vi "TestMathvsWhileLoop.vi"() -> ()   [LabVIEW 2014]
panel:
  out "Math Better?":bool
  out "Maths time":dbl
  out "While loop time":dbl
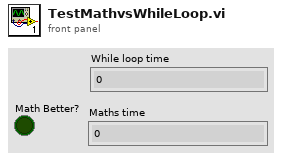
[diagram p1: front panel]
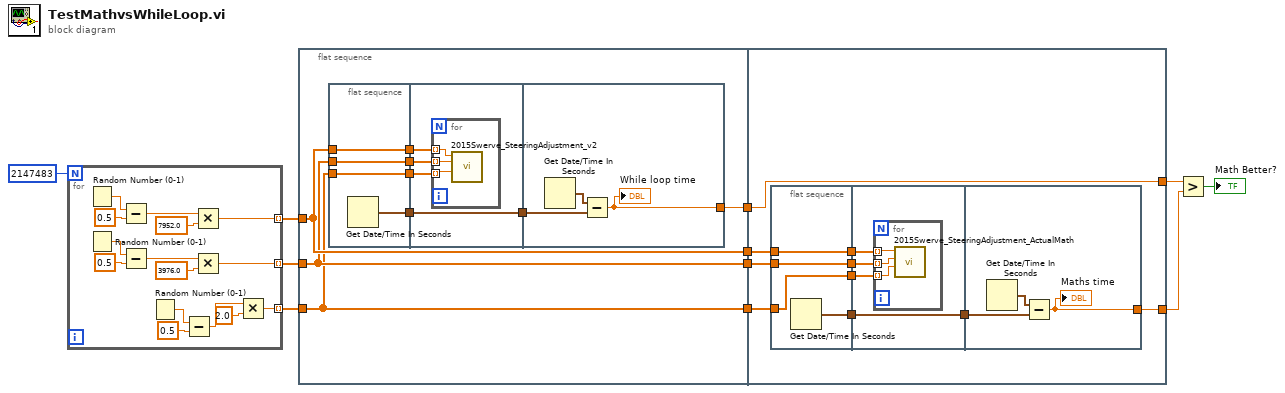
[diagram p0: block diagram]
diagram:
  n1 = for {
    N: 2147483 -> [_]
    tunnel: [w18] -> w8 mode=indexing
    tunnel: [w17] -> w10 mode=indexing
    tunnel: [w12] -> w9 mode=indexing
    n2 = Random Number (0-1)() -> (number: 0 to 1=w26:dbl)
    n3 = Random Number (0-1)() -> (number: 0 to 1=w13:dbl)
    n4 = Subtract(x=w26, y=0.5) -> (x-y=w24:dbl)
    n5 = Subtract(x=w13, y=0.5) -> (x-y=w15:dbl)
    n6 = Random Number (0-1)() -> (number: 0 to 1=w19:dbl)
    n7 = Subtract(x=w19, y=0.5) -> (x-y=w21:dbl)
    n8 = Multiply(x=w24, y=7952.0) -> (x*y=w17:dbl)
    n9 = Multiply(x=w15, y=3976.0) -> (x*y=w12:dbl)
    n10 = Multiply(x=w21, y=2.0) -> (x*y=w18:dbl)
  }
  n11 = flat-sequence {
    tunnel: w10 -> [w29]
    tunnel: w9 -> [w28]
    tunnel: w8 -> [w27]
    tunnel: [w30] -> w5
    tunnel: [w29] -> w4
    tunnel: [w28] -> w3
    tunnel: [w27] -> w2
    tunnel: [w59] -> w7
    tunnel: w5 -> [w59]
    tunnel: w4 -> [w55]
    tunnel: w3 -> [w53]
    tunnel: w2 -> [w52]
    tunnel: [w50] -> w1
    frame #0 {
      n12 = flat-sequence {
        tunnel: [w39] -> w35
        tunnel: w28 -> [w38]
        tunnel: [w38] -> w34
        tunnel: w29 -> [w37]
        tunnel: [w37] -> w33
        tunnel: [w36] -> w32
        tunnel: w27 -> [w36]
        tunnel: w35 -> [w43]
        tunnel: [w43] -> w31
        tunnel: w34 -> [w42]
        tunnel: w33 -> [w41]
        tunnel: w32 -> [w40]
        tunnel: w31 -> [w48]
        tunnel: [w47] -> w30
        frame #0 {
          n13 = Get Date/Time In Seconds() -> (seconds since 1Jan1904=w39:timestamp)
        }
        frame #1 {
          n14 = for {
            tunnel: w42 -> [w45] mode=indexing
            tunnel: w41 -> [w46] mode=indexing
            tunnel: w40 -> [w44] mode=indexing
            n15 = call "2015Swerve_SteeringAdjustment_v2.vi"("Wheel Power"=w44, "Encoder Setpoint"=w45, "Encoder Position"=w46) -> ()  [unwired: 7 in, 2 out]
          }
        }
        frame #2 {
          n16 = Get Date/Time In Seconds() -> (seconds since 1Jan1904=w49:timestamp)
          n17 = Subtract(x=w49, y=w48) -> (x-y=w47:dbl)
          "While loop time" <- w47
        }
      }
    }
    frame #1 {
      n18 = flat-sequence {
        tunnel: [w63] -> w58
        tunnel: [w62] -> w56
        tunnel: w55 -> [w62]
        tunnel: [w61] -> w54
        tunnel: w53 -> [w61]
        tunnel: w52 -> [w60]
        tunnel: [w60] -> w51
        tunnel: w58 -> [w67]
        tunnel: [w67] -> w57
        tunnel: w56 -> [w66]
        tunnel: w54 -> [w65]
        tunnel: w51 -> [w64]
        tunnel: w57 -> [w72]
        tunnel: [w71] -> w50
        frame #0 {
          n19 = Get Date/Time In Seconds() -> (seconds since 1Jan1904=w63:timestamp)
        }
        frame #1 {
          n20 = for {
            tunnel: w66 -> [w70] mode=indexing
            tunnel: w65 -> [w69] mode=indexing
            tunnel: w64 -> [w68] mode=indexing
            n21 = call "2015Swerve_SteeringAdjustment_ActualMath.vi"("Wheel Power"=w68, "Encoder Setpoint"=w69, "Encoder Position"=w70) -> ()  [unwired: 7 in, 2 out]
          }
        }
        frame #2 {
          n22 = Get Date/Time In Seconds() -> (seconds since 1Jan1904=w73:timestamp)
          n23 = Subtract(x=w73, y=w72) -> (x-y=w71:dbl)
          "Maths time" <- w71
        }
      }
    }
  }
  n24 = Greater?(x=w7, y=w1) -> (0:→"Math Better?":bool)
